vi "IntakeToggle-C.vi"(11 "Params":string[][](array[string])) -> ()   [LabVIEW 2020]
uses:
  Framework/Robot Global Data.vi
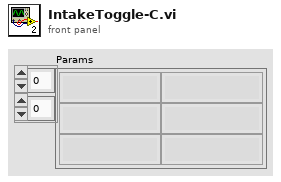
[diagram p1: front panel]
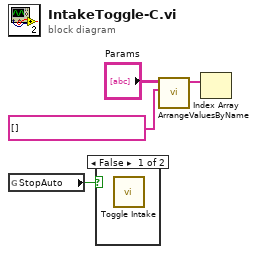
[diagram p0: block diagram]
diagram:
  n1 = global read "Robot Global Data.vi" "StopAuto"() -> (w4:bool)
  n2 = case shown="False" w4 {
    frame False {
      n3 = call "Toggle Intake.vi"() -> ()  [unwired: 11 in, 1 out]
    }
    frame True {
    }
  }
  n4 = call "ArrangeValuesByName.vi"("Names"=string[] [], "Names/Values in"="Params") -> ("Values Out"=w1:string[])  [unwired: 9 in]
  n5 = Index Array(array=w1) -> ()  [unwired: 1 in, 1 out]
